vi "Cryo-Con Get T and H.vi"(8 "error in (no error)":errorcluster, 10 "Private data":T1={"Channels to measure"=[], "Record heater"=FALSE, "Set point"=0.0, "Heater Range"=enum."0.25W", "Control"=FALSE, "Loop type"=enum."Off", "Ramp rate,\n K/min"=1.0, "Control Channel"="A", "P"=0.0, "I"=0.0, "D"=0.0, "Manual %"=0}, 11 "VISA Resource Name":refnum<visa-resource-name>) -> (0 "error out":errorcluster, 1 "data string":string, 2 "Data out":dbl[](array[numeric]), 3 "VISA Resource Name Out":refnum<visa-resource-name>, 4 "Heat %":dbl format="%.2f")   [LabVIEW 2015]
uses:
  Cryo-Con Front Panel Data.ctl
  Cryo-con Heater Ranges.ctl
  Cry-Con Loop Type.ctl
panel:
  # "Temperature Monitor"
  # "Temperature Control"
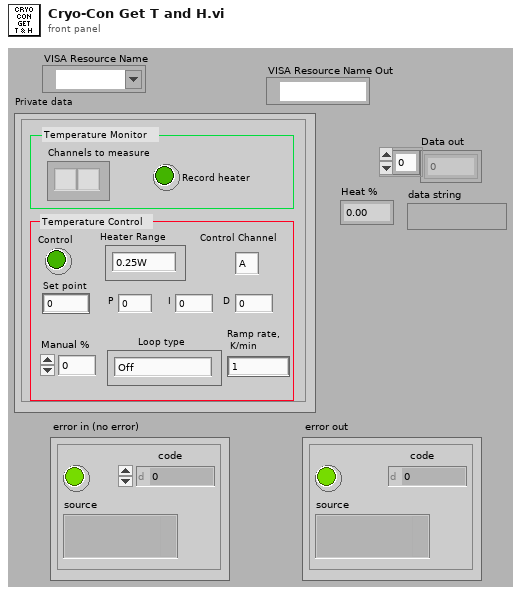
[diagram p1: front panel]
types:
  T1 = typedef "Cryo-Con Front Panel Data.ctl" = cluster{"Channels to measure":string[], "Record heater":bool, "Set point":dbl, "Heater Range":T2, "Control":bool, "Loop type":T3, "Ramp rate,\n K/min":dbl, "Control Channel":string, "P":dbl, "I":dbl, "D":dbl, "Manual %":u16}
  T2 = typedef "Cryo-con Heater Ranges.ctl" = enum16{"25W", "2.5W", "0.25W"}
  T3 = typedef "Cry-Con Loop Type.ctl" = enum16{"Off", "PID", "Manual", "PID Table", "PID Ramp", "PID Table Ramp"}
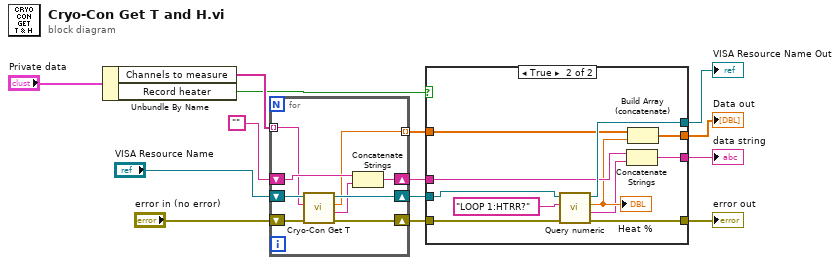
[diagram p0: block diagram]
diagram:
  n1 = Unbundle By Name("Private data") -> ("Channels to measure"=w11:string[], "Record heater"=w9:bool)
  n2 = for {
    shift-right: [w21] -> w6
    shift-left: "VISA Resource Name" -> [w22]
    shift-right: [w23] -> w8
    shift-left: "error in (no error)" -> [w16]
    tunnel: w11 -> [w15] mode=indexing
    tunnel: [w17] -> w2 mode=indexing
    shift-right: [w19] -> w4
    shift-left: "" -> [w20]
    n3 = call "Cryo-Con Get T.vi"("error in (no error)"=w16, "Channel"=w15, "VISA Resource Name"=w22) -> ("error out"=w23:errorcluster, "data string"=w18:string, "Temperature"=w17:dbl, "VISA Resource Name Out"=w21:refnum<visa-resource-name>)  [unwired: 5 in]
    n4 = Concatenate Strings(w20, w18) -> (w19:string)
  }
  n5 = case shown="True" w9 {
    tunnel: w8 -> [w27 w31]
    tunnel: [w27 w38] -> w7
    tunnel: w6 -> [w26 w32]
    tunnel: [w26 w37] -> w5
    tunnel: w4 -> [w25 w36]
    tunnel: [w25 w35] -> w3
    tunnel: w2 -> [w24 w34]
    tunnel: [w24 w33] -> w1
    frame False {
    }
    frame True {
      n6 = call "Query numeric.vi"("Error In"=w31, "Query String"="LOOP 1:HTRR?", "VISA resource name"=w32) -> ("Error Out"=w38:errorcluster, "data string out"=w28:string, "Numeric"=w30:dbl, "VISA resource name out"=w37:refnum<visa-resource-name>)  [unwired: 5 in]
      "Heat %" <- w30
      n7 = Concatenate Strings(w36, w28) -> (w35:string)
      n8 = Build Array (concatenate)(w34, w30) -> (w33:dbl[])
    }
  }
  "error out" <- w7
  "data string" <- w3
  "Data out" <- w1
  "VISA Resource Name Out" <- w5
